vi "Get request ID.vi"(8 "error in (no error)":errorcluster, 10 "message":string) -> (0 "error out":errorcluster, 2 "ID":i32)   [LabVIEW 2020]
uses:
  <vilib>/regexp/Match Regular Expression.xnode
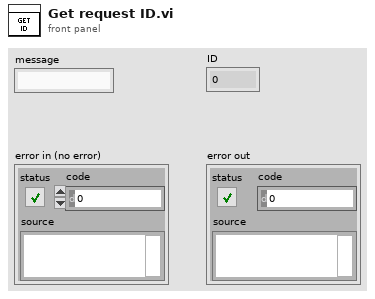
[diagram p1: front panel]
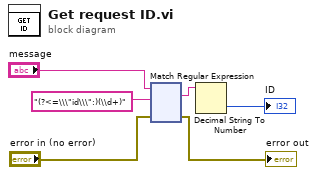
[diagram p0: block diagram]
diagram:
  n1 = xnode "Match Regular Expression"("input string"="message", "regular expression"="(?<=\\\"id\\\":)(\\d+)", "error in"="error in (no error)") -> ("whole match"=w2:string, "error out"=→"error out":errorcluster)  [unwired: 3 in, 3 out]
  n2 = Decimal String To Number(string=w2) -> (number=→"ID":i32)  [unwired: 2 in, 1 out]
